vi "set_TRIG.vi"   [LabVIEW 2011]
doc: "reads the global variables and configurates TRIG1 & TRIG2 accordingly"
uses:
  global.vi
panel:
  # "see block diagram"
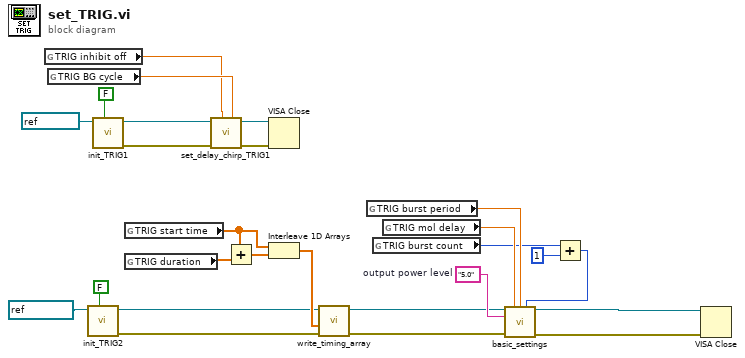
[diagram p0: block diagram]
diagram:
  w25 = "5.0"  # output power level
  n1 = global read "global.vi" "TRIG inhibit off"() -> (w5:dbl)
  n2 = global read "global.vi" "TRIG BG cycle"() -> (w19:dbl)
  n3 = call "init_TRIG2.vi"("reset TRIG"=FALSE, "VISA resource name"=refnum<visa-resource-name> "TRIG2" ("TRIG2 resource name")) -> ("error out"=w12:errorcluster, "VISA resource name out"=w13:refnum<visa-resource-name>)  [unwired: 5 in]
  n4 = call "init_TRIG1.vi"("reset"=FALSE, "VISA resource name"=refnum<visa-resource-name> "TRIG1") -> ("error out"=w17:errorcluster, "VISA resource name out"=w18:refnum<visa-resource-name>)  [unwired: 8 in]
  n5 = global read "global.vi" "TRIG start time"() -> (w15:dbl[])
  n6 = global read "global.vi" "TRIG duration"() -> (w16:dbl[])
  n7 = call "set_delay_chirp_TRIG1.vi"("background period"=w19, "inhibit off"=w5, "error in"=w17, "VISA resource name"=w18) -> ("error out"=w10:errorcluster, "VISA resource name out"=w11:refnum<visa-resource-name>)  [unwired: 6 in]
  n8 = Add(x=w15, y=w16) -> (x+y=w14:dbl[])
  n9 = VISA Close(VISA resource name=w11, error in (no error)=w10) -> ()  [unwired: 1 out]
  n10 = Interleave 1D Arrays(w15, w14) -> (w24:dbl[])
  n11 = call "write_timing_array.vi"("error in"=w12, "delay array"=w24, "VISA resource in"=w13) -> ("error out 2"=w8:errorcluster, "VISA resource out"=w9:refnum<visa-resource-name>)  [unwired: 3 in]
  n12 = global read "global.vi" "TRIG burst period"() -> (w26:dbl)
  n13 = global read "global.vi" "TRIG burst count"() -> (w3:i32)
  n14 = global read "global.vi" "TRIG mol delay"() -> (w4:dbl)
  n15 = Add(x=w3, y=1) -> (x+y=w2:i32)
  n16 = call "basic_settings.vi"("VISA resource name"=w9, "molecular delay"=w4, "burst period (s)"=w26, "burst count"=w2, "power level"=w25, "error in (no error)"=w8) -> ("VISA resource name out"=w7:refnum<visa-resource-name>, "error out"=w6:errorcluster)  [unwired: 8 in]
  n17 = VISA Close(VISA resource name=w7, error in (no error)=w6) -> ()  [unwired: 1 out]
